vi "OCRTraing.vi"() -> ()   [LabVIEW 2019]
uses:
  Controls/OCRMainActParam.ctl
  <vilib>/vision/Image Controls.llb/IMAQ Image.ctl
  SubVI/[Global]lang.font.exp
  <vilib>/vision/NI_Vision_Development_Module.lvlib
panel:
  out "Make TrainedDataLED":bool
  in  "OCR_MakeTrainedData":bool
  out "Training Error":bool
  in  "OCR_Package_Name":string
  in  "OCRMainTab":T1(tab)
  out "TrainBox":bool
  in  "OCR_TrainBox":bool
  out "MakeTrainningBoxLED":bool
  in  "OCR_MakeTrainingBox":bool
  in  "TemplateImageFilePath":path
  out "Extracr Template":T2(plugin-control)
  in  "Training Example number":i32
  in  "OCR_ModifyBox":bool
  in  "OCR_Stop":bool
  out "Origin Image":T2(plugin-control)
  out "Response Message":string[](array[string])
  out "Command Message":string[](array[string])
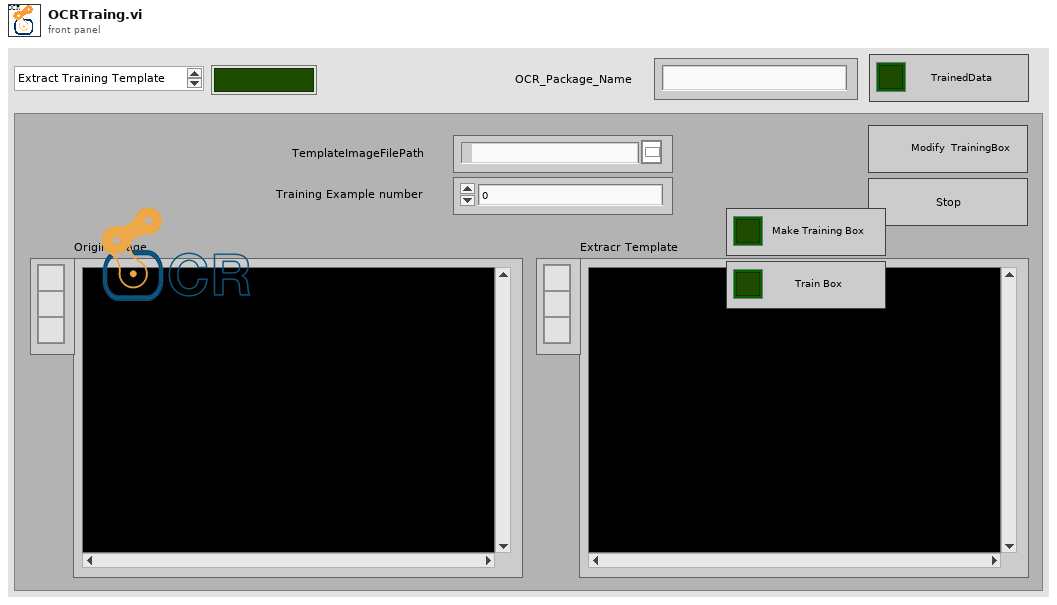
[diagram p1: front panel]
types:
  T1 = enum32{"Extract Training Template", "Message Center"}
  T2 = typedef "IMAQ Image.ctl" = refnum<image>
  T3 = typedef "OCRMainActParam.ctl" = cluster{"OCRMainAction":enum16{"Init", "MakeTrainingBox", "CallJTessBox", "MakeTrainedData", "TrainBox", "LoadImage", "Extract_Save_Image", "MakeTessseractFormat", "Check License", "Stop"}, "OCRMainParam":variant}
  T4 = cluster{"Global Rectangle":i32[], "Contours":cluster{"Contour Type":u32, "ROI Type":u32, "Points":i32[]}[]}
  T5 = enum16{"Init", "MakeTrainingBox", "CallJTessBox", "MakeTrainedData", "TrainBox", "LoadImage", "Extract_Save_Image", "MakeTessseractFormat", "Check License", "Stop"}
  T6 = typedef "Image Type" = u32
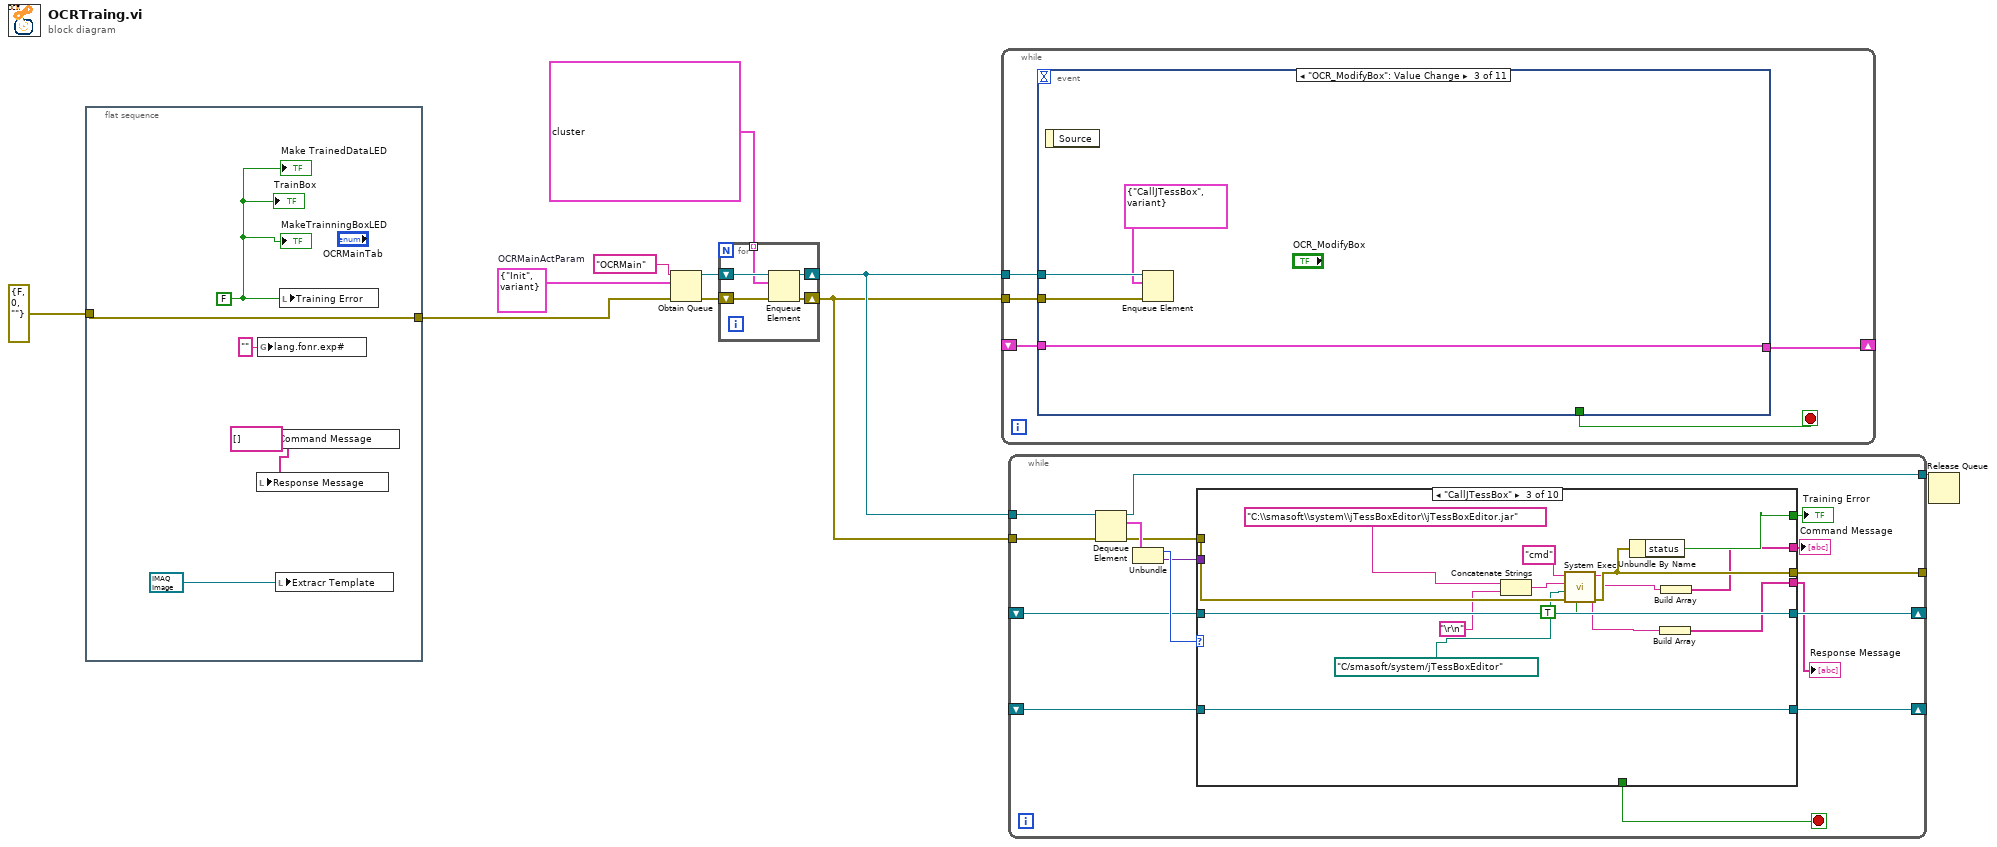
[diagram p0: block diagram]
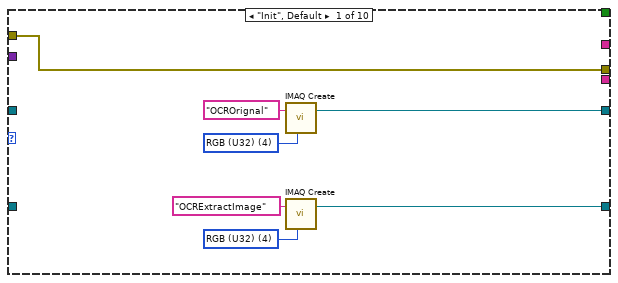
[diagram p2: hidden frame]
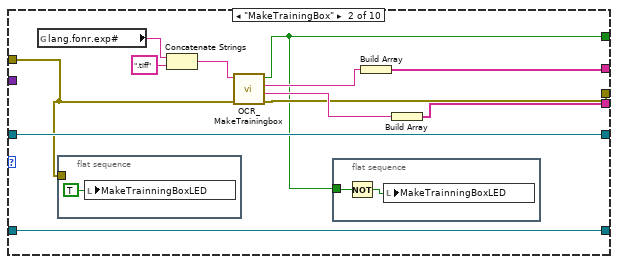
[diagram p3: hidden frame]
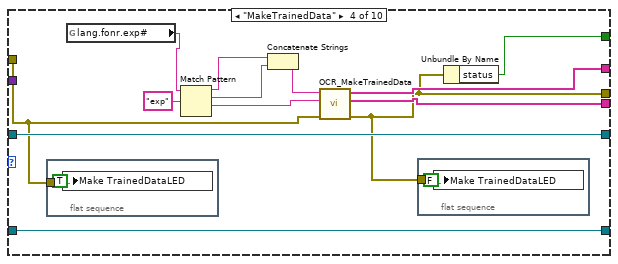
[diagram p4: hidden frame]
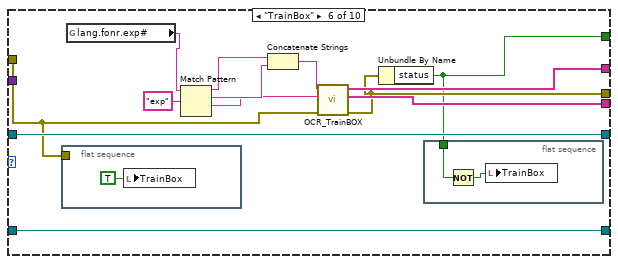
[diagram p6: hidden frame]
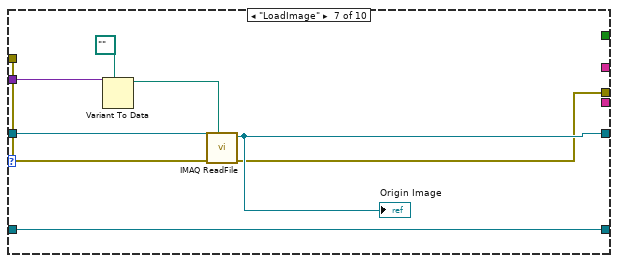
[diagram p7: hidden frame]
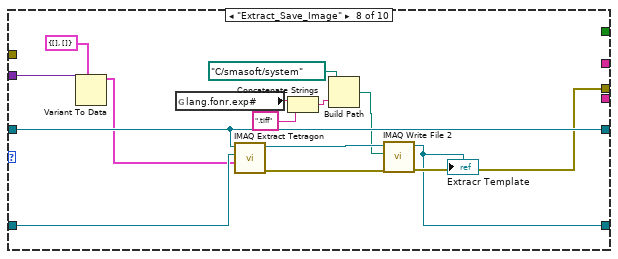
[diagram p8: hidden frame]
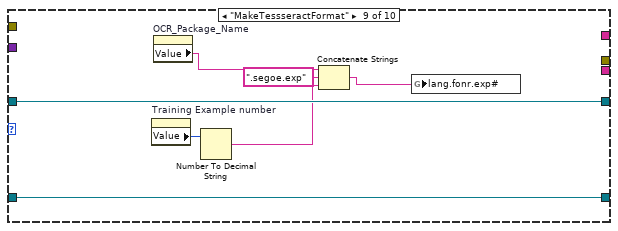
[diagram p9: hidden frame]
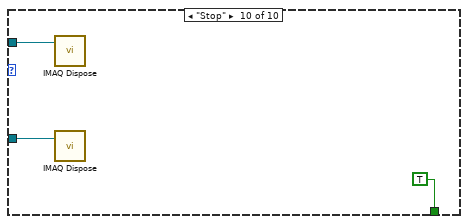
[diagram p10: hidden frame]
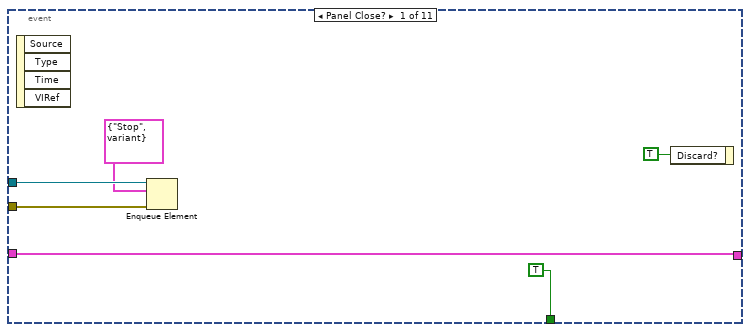
[diagram p11: hidden frame]
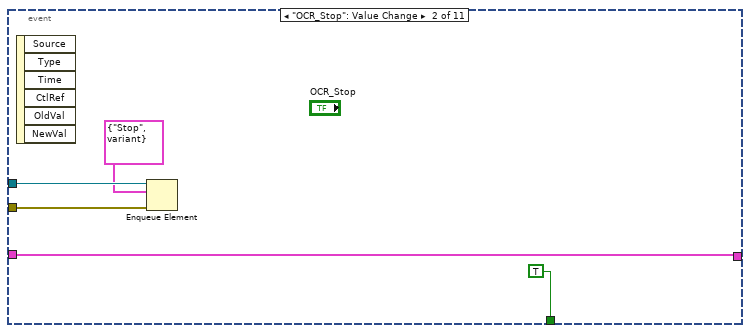
[diagram p12: hidden frame]
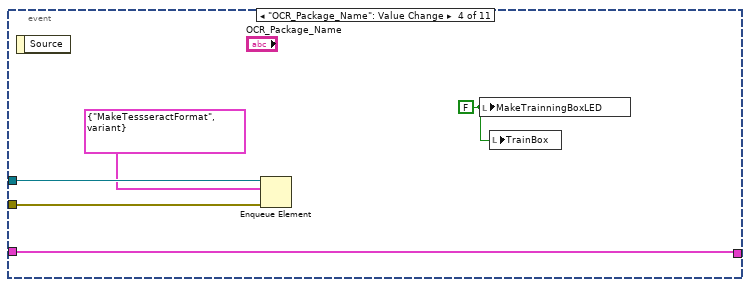
[diagram p13: hidden frame]
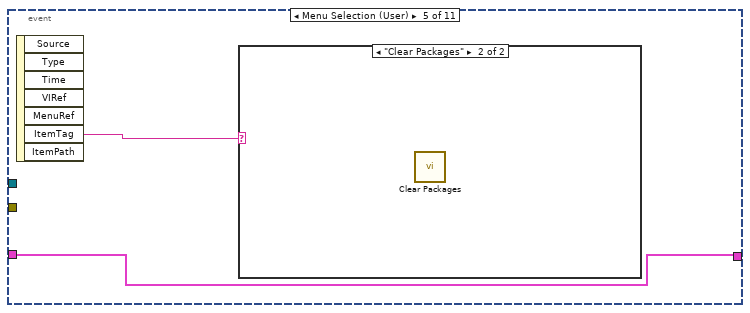
[diagram p14: hidden frame]
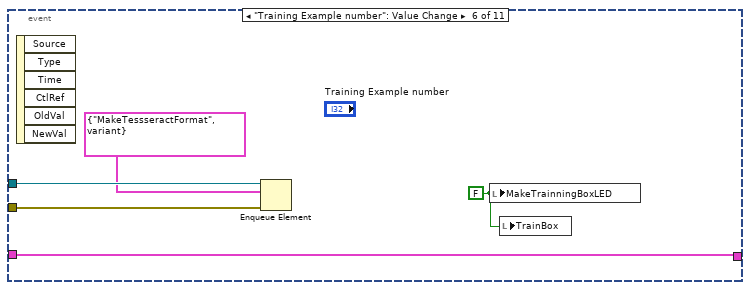
[diagram p16: hidden frame]
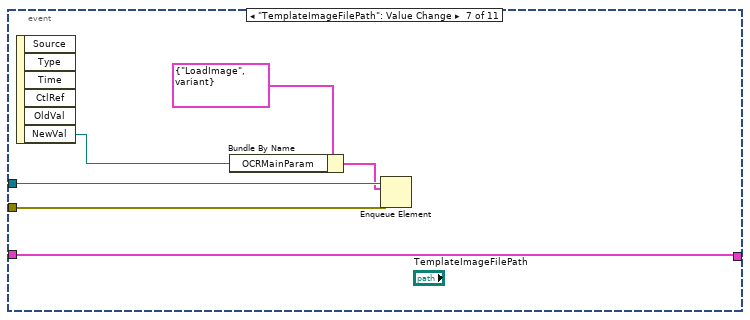
[diagram p17: hidden frame]
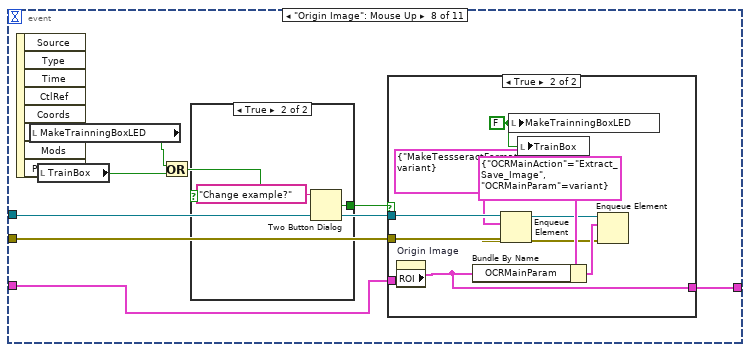
[diagram p18: hidden frame]
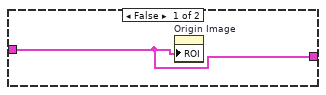
[diagram p19: hidden frame]
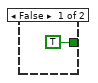
[diagram p20: hidden frame]
diagram:
  w10 = T3 {"OCRMainAction"=enum."Init", "OCRMainParam"=variant}  # OCRMainActParam
  n1 = flat-sequence {
    tunnel: [w15] -> w2
    tunnel: errorcluster {"status"=FALSE, "code"=0, "source"=""} ("error in (no error)") -> [w15]
    frame #0 {
      w12 = string[] [] ("Command")
      w11 = FALSE ("Training Error")
      n2 = local write "Response Message"(w12) -> ()
      n3 = global write "[Global]lang.font.exp" "lang.fonr.exp#"("" ("lang.fonr.exp#")) -> ()
      n4 = local write "Command Message"(w12) -> ()
      n5 = local write "Extracr Template"(T2 refnum ("Extracr Template")) -> ()
      n6 = local write "Training Error"(w11) -> ()
      "TrainBox" <- w11
      "MakeTrainningBoxLED" <- w11
      "Make TrainedDataLED" <- w11
    }
  }
  n7 = Obtain Queue(name (unnamed)="OCRMain" ("element"), element data type=w10, error in (no error)=w2) -> (queue out=w8:refnum<queue>, error out=w5:errorcluster)  [unwired: 2 in, 1 out]
  n8 = for {
    tunnel: T3[] [{"OCRMainAction"=enum."Check License", "OCRMainParam"=variant}, {"OCRMainAction"=enum."Init", "OCRMainParam"=variant}, {"OCRMainAction"=enum."MakeTessseractFormat", "OCRMainParam"=variant}] ("element") -> [w16] mode=indexing
    shift-right: [w19] -> w6
    shift-left: w8 -> [w20]
    shift-right: [w17] -> w4
    shift-left: w5 -> [w18]
    n9 = Enqueue Element(queue=w20, element=w16, error in (no error)=w18) -> (queue out=w19:refnum<queue>, error out=w17:errorcluster)  [unwired: 1 in, 1 out]
  }
  n10 = while {
    tunnel: w6 -> [w25]
    tunnel: w4 -> [w23]
    shift-right: [w22] -> _
    shift-left: _ -> [w21]
    stop <- w24 stop-if-true
    n11 = event shown="[2] \"OCR_ModifyBox\": Value Change" {
      selector: _ -> [_ _ _ _ _ _ _ _ _ _ _]
      dyn-events: _ -> [_ _ _ _ _ _ _ _ _ _ _]
      timeout: _ -> [_ _ _ _ _ _ _ _ _ _ _]
      tunnel: w25 -> [w30 w35 w39 w44 _ w51 w57 w66 w82 w86 w90]
      tunnel: [TRUE TRUE _ _ _ _ _ _ _ _ _] -> w24
      tunnel: w23 -> [w28 w33 w40 w45 _ w52 w58 w65 w83 w87 w91]
      tunnel: [w26 w32 w37 w41 w46 w48 w53 w60 w80 w84 w88] -> w22
      tunnel: w21 -> [w26 w32 w37 w41 w46 w48 w53 w59 w80 w84 w88]
      event Panel Close? {
        n12 = event-data() -> ()  [unwired: 1 in, 4 out]
        n13 = Enqueue Element(queue=w30, element=T3 {"OCRMainAction"=enum."Stop", "OCRMainParam"=variant}, error in (no error)=w28) -> ()  [unwired: 1 in, 3 out]
        n14 = event-data("Discard?"=TRUE) -> ()  [unwired: 1 in, 1 out]
      }
      event "OCR_Stop": Value Change {
        n15 = event-data() -> ()  [unwired: 1 in, 6 out]
        n16 = Enqueue Element(queue=w35, element=T3 {"OCRMainAction"=enum."Stop", "OCRMainParam"=variant}, error in (no error)=w33) -> ()  [unwired: 1 in, 3 out]
      }
      event "OCR_ModifyBox": Value Change {
        n17 = event-data() -> ()  [unwired: 1 in, 1 out]
        n18 = Enqueue Element(queue=w39, element=T3 {"OCRMainAction"=enum."CallJTessBox", "OCRMainParam"=variant}, error in (no error)=w40) -> ()  [unwired: 1 in, 3 out]
      }
      event "OCR_Package_Name": Value Change {
        w42 = FALSE ("MakeTrainningBoxLED")
        n19 = event-data() -> ()  [unwired: 1 in, 1 out]
        n20 = Enqueue Element(queue=w44, element=T3 {"OCRMainAction"=enum."MakeTessseractFormat", "OCRMainParam"=variant}, error in (no error)=w45) -> ()  [unwired: 1 in, 3 out]
        n21 = local write "MakeTrainningBoxLED"(w42) -> ()
        n22 = local write "TrainBox"(w42) -> ()
      }
      event Menu Selection (User) {
        n23 = event-data() -> ("ItemTag"=w47:string)  [unwired: 1 in, 6 out]
        n24 = case shown="\"Clear Packages\"" w47 {
          frame "False", Default {
          }
          frame "Clear Packages" {
            n25 = call "Clear Packages.vi"() -> ()  [unwired: 12 in]
          }
        }
      }
      event "Training Example number": Value Change {
        w49 = FALSE ("MakeTrainningBoxLED")
        n26 = event-data() -> ()  [unwired: 1 in, 6 out]
        n27 = Enqueue Element(queue=w51, element=T3 {"OCRMainAction"=enum."MakeTessseractFormat", "OCRMainParam"=variant}, error in (no error)=w52) -> ()  [unwired: 1 in, 3 out]
        n28 = local write "MakeTrainningBoxLED"(w49) -> ()
        n29 = local write "TrainBox"(w49) -> ()
      }
      event "TemplateImageFilePath": Value Change {
        n30 = event-data() -> ("NewVal"=w55:path)  [unwired: 1 in, 5 out]
        n31 = Bundle By Name(cluster=T3 {"OCRMainAction"=enum."LoadImage", "OCRMainParam"=variant} ("element"), "OCRMainParam"=w55) -> (w54:T3)
        n32 = Enqueue Element(queue=w57, element=w54, error in (no error)=w58) -> ()  [unwired: 1 in, 3 out]
      }
      event "Origin Image": Mouse Up {
        n33 = event-data() -> ()  [unwired: 1 in, 8 out]
        n34 = local read "MakeTrainningBoxLED"() -> (w64:bool)
        n35 = local read "TrainBox"() -> (w63:bool)
        n36 = Or(x=w64, y=w63) -> (x .or. y?=w62:bool)
        n37 = case shown="True" w62 {
          tunnel: [TRUE ("T button?") w78] -> w61
          frame False {
          }
          frame True {
            n38 = Two Button Dialog(message="Change example?") -> (T button?=w78:bool)  [unwired: 2 in]
          }
        }
        n39 = case shown="True" w61 {
          tunnel: w66 -> [_ w76]
          tunnel: w65 -> [_ w72]
          tunnel: [w67 w69] -> w60
          tunnel: w59 -> [w67 _]
          frame False {
            n40 = property on="Origin Image" class="ImageControl"("ROI"=w67) -> ()  [unwired: 2 in, 2 out]
          }
          frame True {
            w68 = FALSE ("MakeTrainningBoxLED")
            n41 = property on="Origin Image" class="ImageControl"() -> ("ROI"=w69:T4)  [unwired: 2 in, 2 out]
            n42 = Bundle By Name(cluster=T3 {"OCRMainAction"=enum."Extract_Save_Image", "OCRMainParam"=variant} ("element"), "OCRMainParam"=w69) -> (w74:T3)
            n43 = Enqueue Element(queue=w76, element=T3 {"OCRMainAction"=enum."MakeTessseractFormat", "OCRMainParam"=variant}, error in (no error)=w72) -> (queue out=w73:refnum<queue>, error out=w71:errorcluster)  [unwired: 1 in, 1 out]
            n44 = local write "MakeTrainningBoxLED"(w68) -> ()
            n45 = local write "TrainBox"(w68) -> ()
            n46 = Enqueue Element(queue=w73, element=w74, error in (no error)=w71) -> ()  [unwired: 1 in, 3 out]
          }
        }
      }
      event "OCR_MakeTrainingBox": Value Change {
        n47 = event-data() -> ()  [unwired: 1 in, 1 out]
        n48 = Enqueue Element(queue=w82, element=T3 {"OCRMainAction"=enum."MakeTrainingBox", "OCRMainParam"=variant}, error in (no error)=w83) -> ()  [unwired: 1 in, 3 out]
      }
      event "OCR_TrainBox": Value Change {
        n49 = event-data() -> ()  [unwired: 1 in, 1 out]
        n50 = Enqueue Element(queue=w86, element=T3 {"OCRMainAction"=enum."TrainBox", "OCRMainParam"=variant}, error in (no error)=w87) -> ()  [unwired: 1 in, 3 out]
      }
      event "OCR_MakeTrainedData": Value Change {
        n51 = event-data() -> ()  [unwired: 1 in, 1 out]
        n52 = Enqueue Element(queue=w90, element=T3 {"OCRMainAction"=enum."MakeTrainedData", "OCRMainParam"=variant}, error in (no error)=w91) -> ()  [unwired: 1 in, 3 out]
      }
    }
  }
  n53 = while {
    tunnel: w6 -> [w107]
    shift-right: [w104] -> _
    shift-left: _ -> [w101]
    shift-right: [w103] -> _
    shift-left: _ -> [w100]
    tunnel: w4 -> [w99]
    tunnel: [w98] -> w7
    tunnel: [w96] -> _
    stop <- w102 stop-if-true
    n54 = Dequeue Element(queue=w107, error in (no error)=w99) -> (queue out=w98:refnum<queue>, element=w106:T3, error out=w97:errorcluster)  [unwired: 1 in, 1 out]
    n55 = Unbundle(w106) -> ("OCRMainAction"=w105:T5, "OCRMainParam"=w95:variant)
    n56 = case shown="\"CallJTessBox\"" w105 {
      tunnel: [w112 w126 w144 w157 w161 w174 w183 w197 w206 _] -> w104
      tunnel: [w111 w125 w143 w156 w160 w173 w185 w191 w205 _] -> w103
      tunnel: [_ _ _ _ _ _ _ _ _ TRUE] -> w102
      tunnel: w101 -> [_ w126 w144 w157 w161 w174 w184 w197 w206 w208]
      tunnel: w100 -> [_ w125 w143 w156 w160 w173 w185 w196 w205 w207]
      tunnel: w97 -> [w110 w117 w142 w146 _ w164 w179 _ _ _]
      tunnel: [w110 w116 w137 w145 _ w163 w178 w193 _ _] -> w96
      tunnel: w95 -> [_ _ _ _ _ _ w180 w199 _ _]
      tunnel: [_ w115 w136 w149 _ w162 _ _ _ _] -> w94
      tunnel: [_ w120 w134 w148 _ w166 _ _ _ _] -> w93
      tunnel: [_ w118 w132 w147 _ w165 _ _ _ _] -> w92
      frame "Init", Default {
        w108 = T6 4 items=["Grayscale (U8)", "Grayscale (I16)", "Grayscale (SGL)", "Complex (CSG)", "RGB (U32)", "HSL (U32)", "RGB (U64)", "Grayscale (U16)"] ("Image Type")
        w109 = T6 4 items=["Grayscale (U8)", "Grayscale (I16)", "Grayscale (SGL)", "Complex (CSG)", "RGB (U32)", "HSL (U32)", "RGB (U64)", "Grayscale (U16)"] ("Image Type")
        n57 = call "IMAQ Create"("Image Name"="OCROrignal", "Image Type"=w109) -> ("New Image"=w112:T2)  [unwired: 3 in, 1 out]
        n58 = call "IMAQ Create"("Image Name"="OCRExtractImage", "Image Type"=w108) -> ("New Image"=w111:T2)  [unwired: 3 in, 1 out]
      }
      frame "MakeTrainingBox" {
        n59 = global read "[Global]lang.font.exp" "lang.fonr.exp#"() -> (w124:string)
        n60 = flat-sequence {
          tunnel: w117 -> [_]
          frame #0 {
            n61 = local write "MakeTrainningBoxLED"(TRUE ("MakeTrainningBoxLED")) -> ()
          }
        }
        n62 = Concatenate Strings(w124, ".tiff" ("string")) -> (w122:string)
        n63 = call "OCR_MakeTrainingbox.vi"("error in (no error)"=w117, "Image Name"=w122) -> ("error out"=w116:errorcluster, "standard error"=w119:string, "standard output"=w121:string, "error"=w115:bool)  [unwired: 6 in]
        n64 = flat-sequence {
          tunnel: w115 -> [w128]
          frame #0 {
            n65 = Not(x=w128) -> (.not. x?=w127:bool)
            n66 = local write "MakeTrainningBoxLED"(w127) -> ()
          }
        }
        n67 = Build Array(w121) -> (w120:string[])
        n68 = Build Array(w119) -> (w118:string[])
      }
      frame "CallJTessBox" {
        n69 = Concatenate Strings("C:\\smasoft\\system\\jTessBoxEditor\\jTessBoxEditor.jar" ("name or relative path"), "\r\n") -> (w139:string)
        n70 = call <vilib>:"System Exec.vi"("run minimized? (F)"=TRUE, "error in (no error)"=w142, "working directory"=path "C:/smasoft/system/jTessBoxEditor", "standard input"=w139, "command line"="cmd") -> ("error out"=w137:errorcluster, "standard error"=w133:string, "standard output"=w135:string)  [unwired: 3 in, 1 out]
        n71 = Unbundle By Name(w137) -> ("status"=w136:bool)
        n72 = Build Array(w133) -> (w132:string[])
        n73 = Build Array(w135) -> (w134:string[])
      }
      frame "MakeTrainedData" {
        n74 = flat-sequence {
          tunnel: w146 -> [_]
          frame #0 {
            n75 = local write "Make TrainedDataLED"(TRUE ("Make TrainedDataLED")) -> ()
          }
        }
        n76 = global read "[Global]lang.font.exp" "lang.fonr.exp#"() -> (w155:string)
        n77 = Match Pattern(string=w155, regular expression="exp") -> (before substring=w153:string, match substring=w152:string, after substring=w151:string)  [unwired: 1 in, 1 out]
        n78 = Concatenate Strings(w153, w152) -> (w150:string)
        n79 = call "OCR_MakeTrainedData.vi"("error in (no error)"=w146, "exp#"=w151, "lang.font.exp"=w150) -> ("error out"=w145:errorcluster, "standard error"=w147:string[], "standard output"=w148:string[])  [unwired: 6 in]
        n80 = flat-sequence {
          tunnel: w145 -> [_]
          frame #0 {
            n81 = local write "Make TrainedDataLED"(FALSE ("Make TrainedDataLED")) -> ()
          }
        }
        n82 = Unbundle By Name(w145) -> ("status"=w149:bool)
      }
      frame "Check License" {
      }
      frame "TrainBox" {
        n83 = flat-sequence {
          tunnel: w164 -> [_]
          frame #0 {
            n84 = local write "TrainBox"(TRUE ("TrainBox")) -> ()
          }
        }
        n85 = global read "[Global]lang.font.exp" "lang.fonr.exp#"() -> (w172:string)
        n86 = Match Pattern(string=w172, regular expression="exp") -> (before substring=w170:string, match substring=w169:string, after substring=w168:string)  [unwired: 1 in, 1 out]
        n87 = Concatenate Strings(w170, w169) -> (w167:string)
        n88 = call "OCR_TrainBOX.vi"("error in (no error)"=w164, "exp#"=w168, "lang.font.exp"=w167) -> ("error out"=w163:errorcluster, "standard error"=w165:string[], "standard output"=w166:string[])  [unwired: 6 in]
        n89 = Unbundle By Name(w163) -> ("status"=w162:bool)
        n90 = flat-sequence {
          tunnel: w162 -> [w175]
          frame #0 {
            n91 = Not(x=w175) -> (.not. x?=w176:bool)
            n92 = local write "TrainBox"(w176) -> ()
          }
        }
      }
      frame "LoadImage" {
        n93 = Variant To Data(type=path "" ("TemplateImageFilePath"), Variant=w180) -> (data=w181:path)  [unwired: 1 in, 1 out]
        n94 = call "IMAQ ReadFile"("File Path"=w181, "error in (no error)"=w179, "Image"=w184) -> ("error out"=w178:errorcluster, "Image Out"=w183:T2)  [unwired: 4 in, 3 out]
        "Origin Image" <- w183
      }
      frame "Extract_Save_Image" {
        n95 = Variant To Data(type=T4 {"Global Rectangle"=[], "Contours"=[]} ("ROI"), Variant=w199) -> (data=w195:T4)  [unwired: 1 in, 1 out]
        n96 = global read "[Global]lang.font.exp" "lang.fonr.exp#"() -> (w189:string)
        n97 = call-poly "IMAQ Extract Tetragon"("ROI Descriptor"=w195, "Image Dst"=w196, "Image Src"=w197) -> ("error out"=w194:errorcluster, "Image Dst Out"=w192:T2)  [unwired: 7 in]
        n98 = Concatenate Strings(w189, ".tiff" ("string")) -> (w187:string)
        n99 = Build Path(base path=path "C:/smasoft/system", name or relative path=w187) -> (appended path=w188:path)
        n100 = call-poly "IMAQ Write File 2"("error in (no error)"=w194, "File Path"=w188, "Image"=w192) -> ("error out"=w193:errorcluster, "Image Out (duplicate)"=w191:T2)  [unwired: 7 in]
        "Extracr Template" <- w191
      }
      frame "MakeTessseractFormat" {
        n101 = property on="Training Example number" class="DigNum (strict)"() -> ("Value"=w204:i32)  [unwired: 2 in, 2 out]
        n102 = property on="OCR_Package_Name" class="Str"() -> ("Value"=w203:string)  [unwired: 2 in, 2 out]
        n103 = Number To Decimal String(number=w204) -> (decimal integer string=w201:string)  [unwired: 1 in]
        n104 = Concatenate Strings(w203, ".segoe.exp" ("string"), w201) -> (w200:string)
        n105 = global write "[Global]lang.font.exp" "lang.fonr.exp#"(w200) -> ()
      }
      frame "Stop" {
        n106 = call "IMAQ Dispose"("Image"=w208) -> ()  [unwired: 5 in, 1 out]
        n107 = call "IMAQ Dispose"("Image"=w207) -> ()  [unwired: 5 in, 1 out]
      }
    }
    "Training Error" <- w94
    "Response Message" <- w92
    "Command Message" <- w93
  }
  n108 = Release Queue(queue=w7) -> ()  [unwired: 2 in, 3 out]
